vi "CAN wait.vi"(8 "error in":errorcluster, 9 "Timeout":i32=1000 format="%d ms", 10 "COB-ID":u32 format="%.0x", 11 "CANopen in":refnum<class "CANopen.lvclass">) -> (0 "error out":errorcluster, 1 "Timed Out?":bool, 3 "CANopen out":refnum<class "CANopen.lvclass">)   [LabVIEW 2026, in "canopen_.lvlib" / "CANopen.lvclass"]
doc: "Waits until a specific COB-ID is sent or a specific timeout is elapsed. This VI is <B>blocking</B>!"
uses:
  CANopen.lvclass
  CANopen.lvclass/CANopen.ctl
panel:
  out "Notification":cluster{"Time Stamp":timestamp, "Data":u8[]}
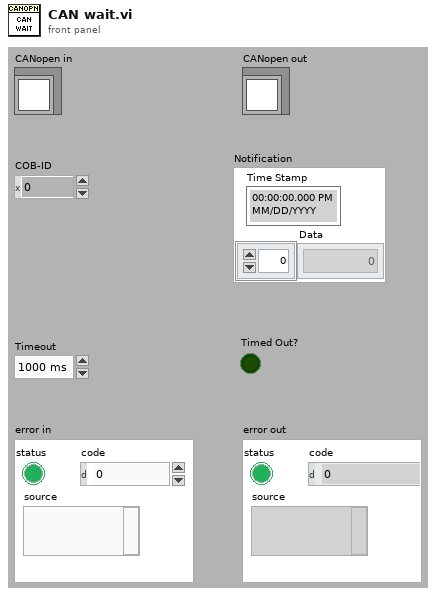
[diagram p1: front panel]
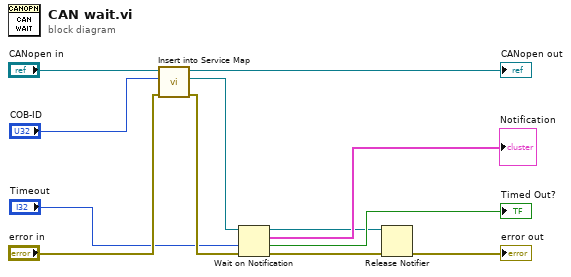
[diagram p0: block diagram]
diagram:
  n1 = call "Insert into Service Map.vi"("error in"="error in", "COB-ID"="COB-ID", "CANopen in"="CANopen in") -> ("error out"=w8:errorcluster, "Notifier"=w7:refnum<notifier>, "CANopen out"=→"CANopen out":refnum<class "CANopen.lvclass">)  [unwired: 6 in]
  n2 = Wait on Notification(notifier=w7, timeout in ms (-1)="Timeout", error in (no error)=w8) -> (notifier out=w1:refnum<notifier>, notification=→"Notification":cluster{"Time Stamp":timestamp, "Data":u8[]}, timed out?=→"Timed Out?":bool, error out=w3:errorcluster)  [unwired: 1 in]
  n3 = Release Notifier(notifier=w1, error in (no error)=w3) -> (error out=→"error out":errorcluster)  [unwired: 1 in, 2 out]
